vi "Framework.Set Transceivers.vi"(10 "Transceivers":refnum<class "Transceiver.lvclass">[](array[class]), 11 "Framework in":refnum<class "Framework.lvclass">) -> (3 "Framework out":refnum<class "Framework.lvclass">)   [LabVIEW 2017, in "DSF.Engine.lvlib" / "Framework.lvclass"]
uses:
  Framework.lvclass
  Transceiver/Transceiver.lvclass
  Framework.lvclass/Framework.ctl
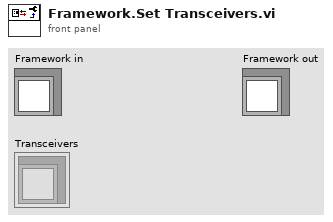
[diagram p1: front panel]
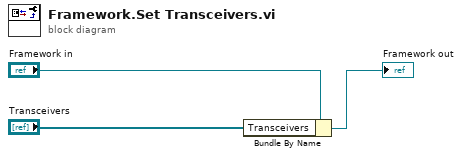
[diagram p0: block diagram]
diagram:
  n1 = Bundle By Name(cluster="Framework in", "Transceivers"="Transceivers") -> (→"Framework out":refnum<class "Framework.lvclass">)
